vi "Sub Topics.vi"() -> ()   [LabVIEW 2014]
uses:
  <userlib>/ROS for LabVIEW Software/ROS/Code/Console/Servers/ServerSubs/TopicDef.ctl
  <userlib>/ROS for LabVIEW Software/ROS/Code/SubVIs/_ROSDirection.ctl
  <userlib>/ROS for LabVIEW Software/ROS/Code/_ROSDefinition.vi
  <userlib>/ROS for LabVIEW Software/ROS/MessageParsing/std_msgs/subs/parse_string_scalar.vi
  <userlib>/ROS for LabVIEW Software/ROS/MessageParsing/std_msgs/subs/parse_float32_scalar.vi
panel:
  out "number 2":i32[](array[numeric])
  out "number":sgl
  in  "ROS Master":string="172.16.0.10:11311"
  out "I heard:":string
  out "error out":errorcluster
  in  "stop":bool
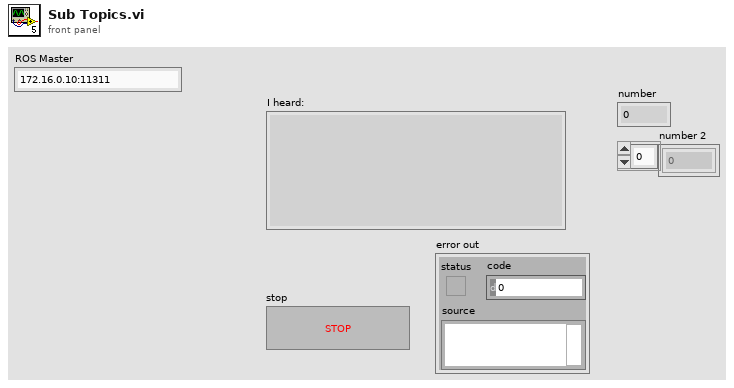
[diagram p1: front panel]
types:
  T1 = typedef "TopicDef.ctl" = cluster{"Topic":string, "Type":string, "Action":T2, "Update (ms)":u16, "queue size":u16}
  T2 = typedef "_ROSDirection.ctl" = enum16{"Node", "Publisher", "Subscriber", "ServiceClient", "ServiceProvider"}
  T3 = typedef "_ROSControl.ctl" = cluster{"topic port":u16, "Node":string, "topic":string, "type":string, "node port":u16, "error ":errorcluster, "Direction":T2, "Update (ms)":u16, "FIFO size":u16}
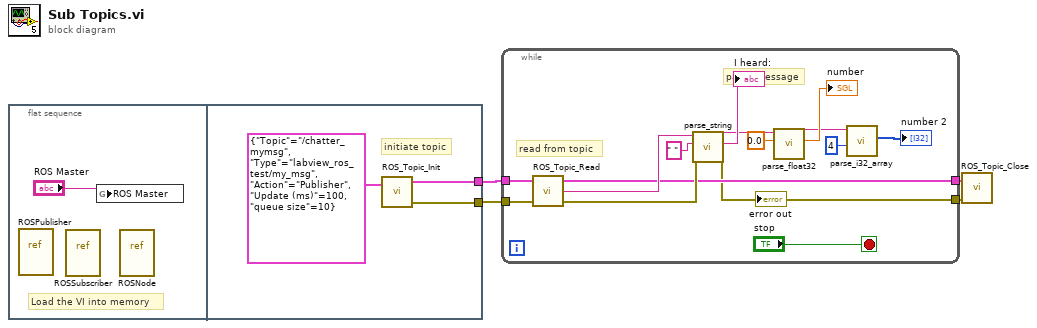
[diagram p0: block diagram]
diagram:
  n1 = flat-sequence {
    tunnel: [w7] -> w2
    tunnel: [w6] -> w1
    frame #0 {
      # "Load the VI into memory"
      n2 = vi-ref <userlib>:"ROSPublisher.vi"() -> ()  [unwired: 1 out]
      n3 = vi-ref <userlib>:"ROSSubscriber.vi"() -> ()  [unwired: 1 out]
      n4 = global write "_ROSDefinition.vi" "ROS Master"("ROS Master") -> ()
      n5 = vi-ref <userlib>:"ROSNode.vi"() -> ()  [unwired: 1 out]
    }
    frame #1 {
      # "initiate topic"
      n6 = call <userlib>:"ROS_Topic_Init.vi"("Definitions"=T1 {"Topic"="/chatter_mymsg", "Type"="labview_ros_test/my_msg", "Action"=enum."Publisher", "Update (ms)"=100, "queue size"=10}) -> ("ROS out"=w7:T3, "error out"=w6:errorcluster)  [unwired: 2 in]
    }
  }
  n7 = while {
    tunnel: w2 -> [w23]
    tunnel: w1 -> [w19]
    tunnel: [w16] -> w4
    tunnel: [w15] -> w3
    stop <- "stop" stop-if-true
    # "parse message"
    # "read from topic"
    n8 = call <userlib>:"ROS_Topic_Read.vi"("error in (no error)"=w19, "ROS in"=w23) -> ("error out"=w18:errorcluster, "Reply"=w22:string, "ROS out"=w16:T3)  [unwired: 1 in]
    n9 = call-poly <userlib>:"parse_string.vi"("error in"=w18, "type"=" ", "msg in"=w22) -> ("error out"=w15:errorcluster, "string"=→"I heard:":string, "msg out"=w14:string)  [unwired: 2 in]
    "error out" <- w15
    n10 = call-poly <userlib>:"parse_float32.vi"("type"=sgl 0.0, "msg in"=w14) -> ("number"=→"number":sgl, "msg out"=w11:string)  [unwired: 3 in, 1 out]
    n11 = call <userlib>:"parse_i32_array.vi"("Array Size"=4, "msg in"=w11) -> ("number"=→"number 2":i32[])  [unwired: 3 in, 2 out]
  }
  n12 = call <userlib>:"ROS_Topic_Close.vi"("error in"=w3, "ROS in"=w4) -> ()  [unwired: 2 in, 1 out]
